vi "globalneZmienneInterfejsu.vi"(8 "Akcja":T2, 11 "globalneZmienneInterfejsuWejscie":T1) -> (3 "globalneZmienneInterfejsuWyjscie":T1)   [LabVIEW 2014]
uses:
  glownaMaszynaStanowVIs/AkcjaGFV.ctl
  globalneZmienneInterfejsuVIs/globalneZmienneInterfejsuParametry.ctl
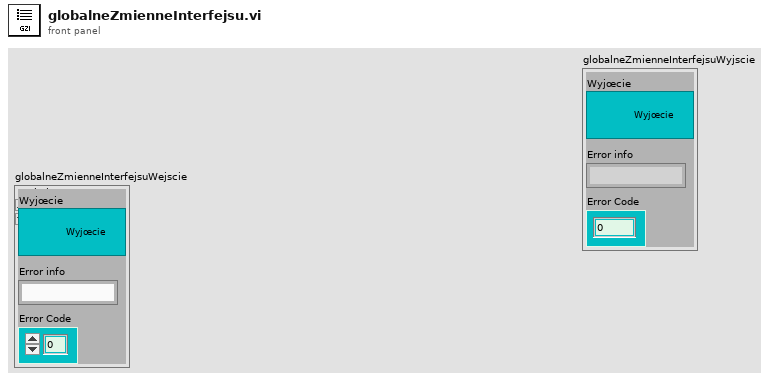
[diagram p1: front panel]
types:
  T1 = typedef "globalneZmienneInterfejsuParametry.ctl" = cluster{"Error info":string, "Wyjœcie":bool, "Error Code":i32}
  T2 = typedef "AkcjaGFV.ctl" = enum16{"Czytaj", "Zapisz", "Reset"}
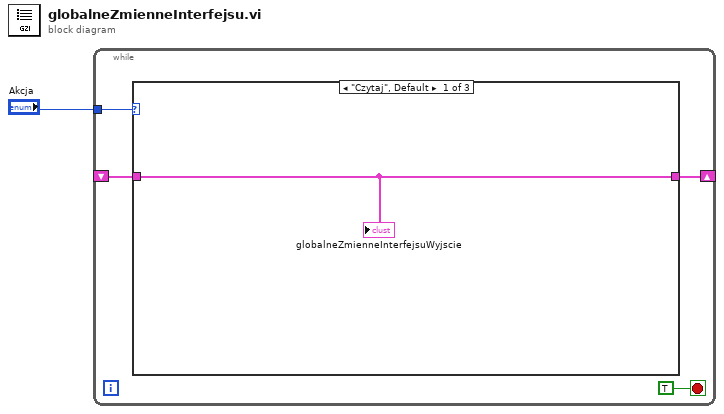
[diagram p0: block diagram]
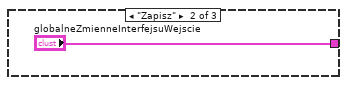
[diagram p2: hidden frame]
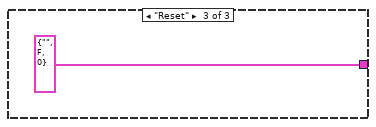
[diagram p3: hidden frame]
diagram:
  n1 = while {
    tunnel: "Akcja" -> [w4]
    shift-right: [w3] -> _
    shift-left: _ -> [w2]
    stop <- TRUE stop-if-true
    n2 = case shown="\"Czytaj\", Default" w4 {
      tunnel: [w6 "globalneZmienneInterfejsuWejscie" T1 {"Error info"="", "Wyjœcie"=FALSE, "Error Code"=0} ("globalneZmienneInterfejsuParametry")] -> w3
      tunnel: w2 -> [w6 _ _]
      frame "Czytaj", Default {
        "globalneZmienneInterfejsuWyjscie" <- w6
      }
      frame "Zapisz" {
      }
      frame "Reset" {
      }
    }
  }
